vi "dfd_Calculate Size TF Polynomial.vi"(4 "alignment(left, top)":T2, 5 "format string":string="%.0f", 6 "rendering options":T1, 7 "Fonts Input":T3(array[cluster]), 8 "variable":string="s", 9 "origin":cluster{"x":i16, "y":i16}={"x"=60, "y"=30}, 10 "coefficients":dbl[](array[numeric])=[0.0, 1.0] format="%.2f") -> (2 "text rect":T4={"left"=60, "top"=30, "right"=68, "bottom"=43})   [LabVIEW 2017, in "NI_DigFilter_Process.lvlib"]
doc: "This VI allow to render Polynomials in Picture Control in ascending/descending order of coefficients, ascending/descending order of polynomial and with negative coefficients."
uses:
  <vilib>/addons/Digital Filter Design/NI_DigFilter_Process.lvlib
panel:
  in  "Fonts Defaut":T3(array[cluster])=[{"Font Name:"="Tahoma", "Size"=13, "Strikeout?"=FALSE, "Italic?"=FALSE, "Underline?"=FALSE, "Outline?"=FALSE, "Shadow?"=FALSE, "Bold?"=FALSE}, {"Font Name:"="Tahoma", "Size"=13, "Strikeout?"=FALSE, "Italic?"=FALSE, "Underline?"=FALSE, "Outline?"=FALSE, "Shadow?"=FALSE, "Bold?"=FALSE}, {"Font Name:"="Tahoma", "Size"=11, "Strikeout?"=FALSE, "Italic?"=FALSE, "Underline?"=FALSE, "Outline?"=FALSE, "Shadow?"=FALSE, "Bold?"=FALSE}]
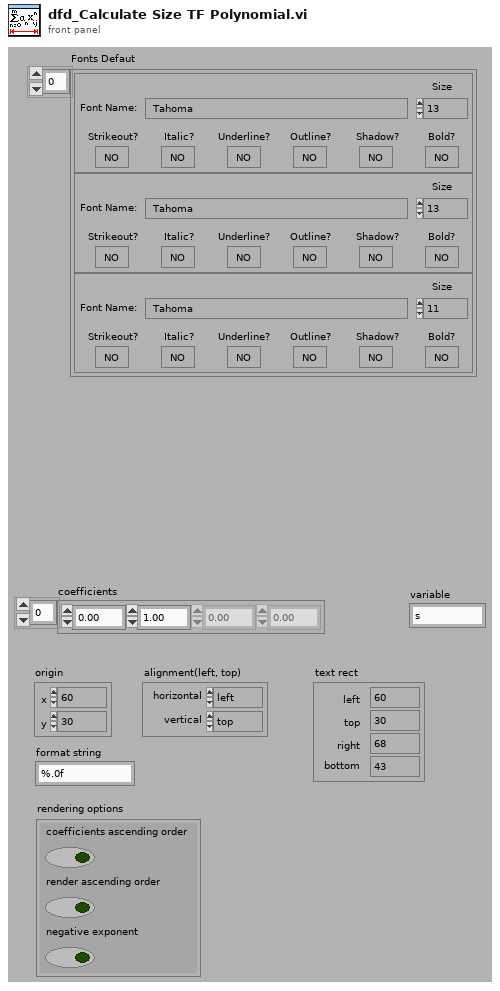
[diagram p1: front panel]
types:
  T1 = cluster{"coefficients ascending order":bool, "render ascending order":bool, "negative exponent":bool}
  T2 = cluster{"horizontal":enum16{"left", "center", "right"}, "vertical":enum16{"top", "center", "bottom"}}
  T3 = cluster{"Font Name:":string, "Size":i16, "Strikeout?":bool, "Italic?":bool, "Underline?":bool, "Outline?":bool, "Shadow?":bool, "Bold?":bool}[]
  T4 = cluster{"left":i16, "top":i16, "right":i16, "bottom":i16}
  T5 = enum16{"User-specified Font", "Application Font", "System Font", "Dialog Font"}
  T6 = cluster{"Font Name:":string, "Size":i16, "Strikeout?":bool, "Italic?":bool, "Underline?":bool, "Outline?":bool, "Shadow?":bool, "Bold?":bool}
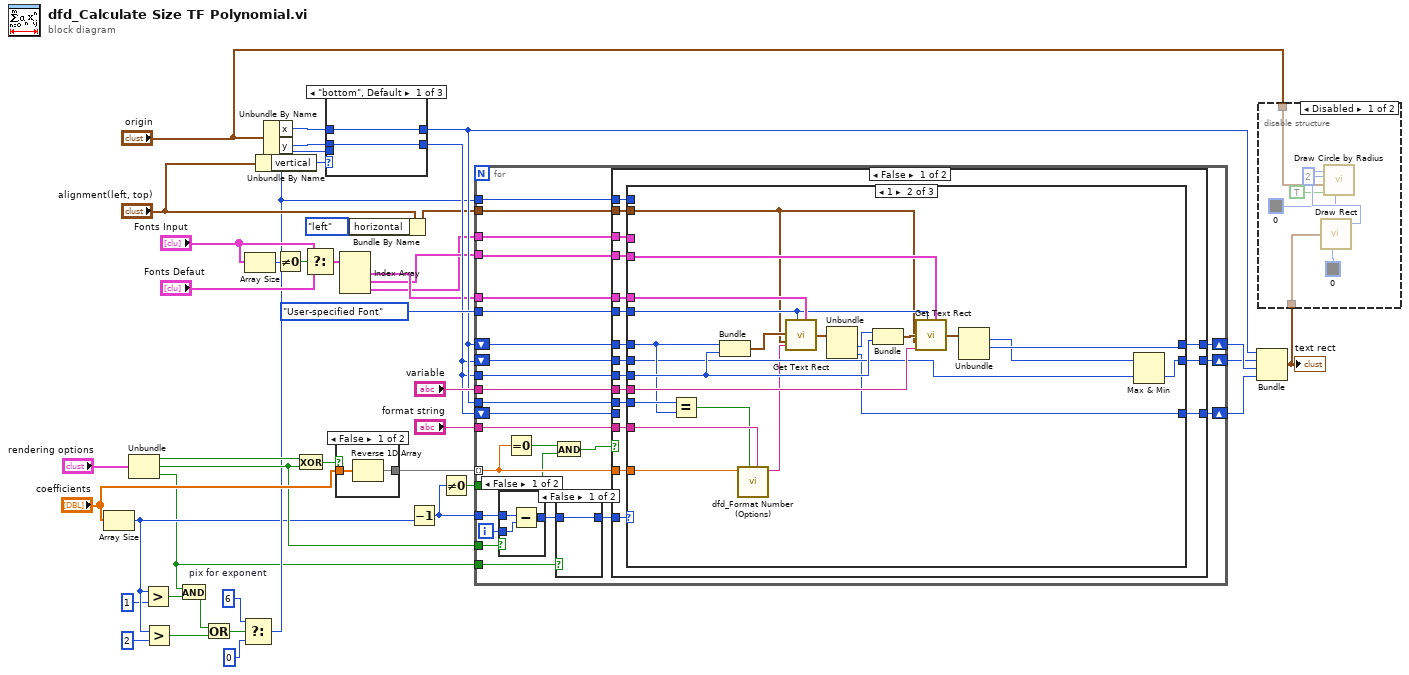
[diagram p0: block diagram]
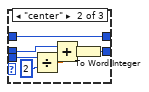
[diagram p3: hidden frame]
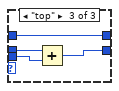
[diagram p4: hidden frame]
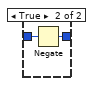
[diagram p6: hidden frame]
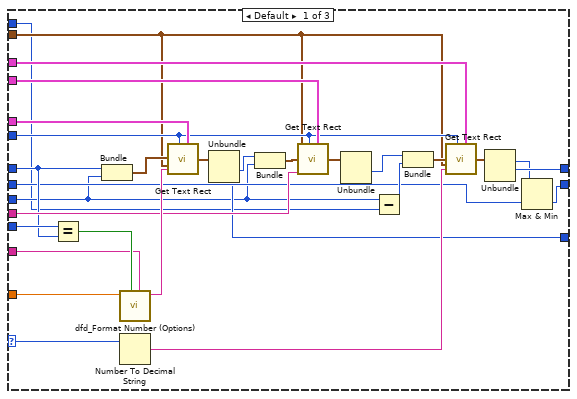
[diagram p8: hidden frame]
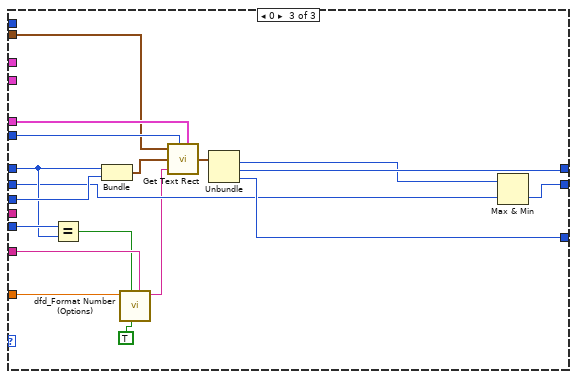
[diagram p9: hidden frame]
diagram:
  w12 = i16 6  # pix for exponent
  n1 = Array Size(array="coefficients") -> (size(s)=w5:i32)
  n2 = Unbundle("rendering options") -> ("coefficients ascending order"=w15:bool, "render ascending order"=w14:bool, "negative exponent"=w3:bool)
  n3 = Greater?(x=w5, y=1) -> (0:w2:bool)
  n4 = Greater?(x=w5, y=2) -> (0:w7:bool)
  n5 = And(x=w3, y=w2) -> (x .and. y?=w1:bool)
  n6 = Or(x=w1, y=w7) -> (x .or. y?=w6:bool)
  n7 = Select(t=w12, s=w6, f=i16 0) -> (s? t:f=w10:i16)
  n8 = Array Size(array="Fonts Input") -> (size(s)=w33:i32)
  n9 = Unbundle By Name("alignment(left, top)") -> ("vertical"=w23:enum16{"top", "center", "bottom"})
  n10 = Unbundle By Name("origin") -> ("x"=w22:i16, "y"=w21:i16)
  n11 = Not Equal To 0?(x=w33) -> (x != 0?=w34:bool)
  n12 = Exclusive Or(1:w14, 2:w15) -> (0:w25:bool)
  n13 = Select(t="Fonts Input", s=w34, f="Fonts Defaut") -> (s? t:f=w31:T3)
  n14 = case shown="\"bottom\", Default" w23 {
    tunnel: [w45 w52 w56] -> w38
    tunnel: [w44 w46 w54] -> w35
    tunnel: w22 -> [w45 w52 w56]
    tunnel: w21 -> [w44 w51 w55]
    tunnel: w10 -> [_ w49 w53]
    frame "bottom", Default {
    }
    frame "center" {
      n15 = Divide(x=w49, y=i16 2) -> (x/y=w47:dbl)
      n16 = Add(x=w51, y=w47) -> (x+y=w50:dbl)
      n17 = To Word Integer(number=w50) -> (16bit integer=w46:i16)
    }
    frame "top" {
      n18 = Add(x=w55, y=w53) -> (x+y=w54:i16)
    }
  }
  n19 = case shown="False" w25 {
    tunnel: "coefficients" -> [w58 w59]
    tunnel: [w57 w59] -> w36
    frame False {
      n20 = Reverse 1D Array(array=w58) -> (reversed array=w57:dbl[])
    }
    frame True {
    }
  }
  n21 = Index Array(array=w31) -> (element #1=w29:T6, element #2=w28:T6, element #3=w27:T6)  [unwired: 3 in]
  n22 = Bundle By Name(cluster="alignment(left, top)", "horizontal"=enum16{"left", "center", "right"}."left") -> (w19:T2)
  n23 = Decrement(x=w5) -> (x-1=w9:i32)
  n24 = Not Equal To 0?(x=w9) -> (x != 0?=w8:bool)
  n25 = for {
    tunnel: w36 -> [w68] mode=indexing
    tunnel: "variable" -> [w85]
    shift-right: [w83] -> w41
    shift-left: w38 -> [w84]
    tunnel: w35 -> [w82]
    tunnel: w29 -> [w81]
    tunnel: w27 -> [w80]
    tunnel: w28 -> [w79]
    tunnel: w38 -> [w78]
    tunnel: w9 -> [w76]
    shift-right: [w74] -> w40
    shift-left: w35 -> [w75]
    tunnel: T5."User-specified Font" ("desired font(Application)") -> [w73]
    shift-right: [w72] -> w37
    shift-left: w35 -> [w71]
    tunnel: "format string" -> [w70]
    tunnel: w19 -> [w69]
    tunnel: w14 -> [w67]
    tunnel: w3 -> [w64]
    tunnel: w10 -> [w63]
    tunnel: w8 -> [w61]
    i -> [w77]
    n26 = case shown="False" w67 {
      tunnel: w77 -> [w91 w92]
      tunnel: w76 -> [w90 _]
      tunnel: [w89 w92] -> w66
      frame False {
        n27 = Subtract(x=w90, y=w91) -> (x-y=w89:i32)
      }
      frame True {
      }
    }
    n28 = Equal To 0?(x=w68) -> (x = 0?=w60:bool)
    n29 = And(x=w60, y=w61) -> (x .and. y?=w62:bool)
    n30 = case shown="False" w64 {
      tunnel: [w86 w87] -> w65
      tunnel: w66 -> [w86 w88]
      frame False {
      }
      frame True {
        n31 = Negate(x=w88) -> (-x=w87:i32)
      }
    }
    n32 = case shown="False" w62 {
      tunnel: w85 -> [w109 _]
      tunnel: w84 -> [w108 w182]
      tunnel: [w107 w182] -> w83
      tunnel: w68 -> [w106 _]
      tunnel: w82 -> [w105 _]
      tunnel: w81 -> [w104 _]
      tunnel: w80 -> [w103 _]
      tunnel: w79 -> [w102 _]
      tunnel: w78 -> [w101 _]
      tunnel: w65 -> [w100 _]
      tunnel: w75 -> [w99 w181]
      tunnel: [w98 w181] -> w74
      tunnel: w73 -> [w97 _]
      tunnel: [w96 w180] -> w72
      tunnel: w71 -> [_ w180]
      tunnel: w70 -> [w95 _]
      tunnel: w69 -> [w94 _]
      tunnel: w63 -> [w93 _]
      frame False {
        n33 = case shown="1" w100 {
          selector: w100 -> [w111 _ _]
          tunnel: w109 -> [w125 w153 _]
          tunnel: w108 -> [w123 w151 w174]
          tunnel: [w121 w150 w173] -> w107
          tunnel: w106 -> [w113 w141 w164]
          tunnel: w105 -> [w112 w157 w176]
          tunnel: w104 -> [w132 w159 w177]
          tunnel: w103 -> [w133 _ _]
          tunnel: w102 -> [w128 w155 _]
          tunnel: w101 -> [w124 w152 w175]
          tunnel: w99 -> [w120 w149 w169]
          tunnel: [w118 w148 w167] -> w98
          tunnel: w97 -> [w117 w147 w172]
          tunnel: [w116 w146 w171] -> w96
          tunnel: w95 -> [w115 w143 w166]
          tunnel: w94 -> [w114 w145 w170]
          tunnel: w93 -> [w110 _ _]
          frame Default {
            n34 = Equal?(x=w124, y=w123) -> (x = y?=w122:bool)
            n35 = Bundle("x"=w123, "y"=w112) -> (w137:cluster{"x":i16, "y":i16})  [unwired: 1 out]
            n36 = call <vilib>:"dfd_Format Number (Options).vi"("format string"=w115, "Is Higher Coeffiecient?"=w122, "Coefficient"=w113) -> ("String Coefficient"=w139:string)  [unwired: 1 in, 7 out]
            n37 = Number To Decimal String(number=w111) -> (decimal integer string=w135:string)  [unwired: 1 out]
            n38 = call <vilib>:"Get Text Rect.vi"("alignment(left, top)"=w114, "desired font(Application)"=w117, "origin(0,0)"=w137, "text"=w139, "[user-specified font]"=w132) -> ("rect"=w138:T4)  [unwired: 1 in, 3 out]
            n39 = Unbundle(w138) -> ("right"=w127:i16, "bottom"=w116:i16)  [unwired: 2 out]
            n40 = Bundle("right"=w127, "y"=w112) -> (w131:cluster{"right":i16, "y":i16})  [unwired: 1 out]
            n41 = call <vilib>:"Get Text Rect.vi"("alignment(left, top)"=w114, "desired font(Application)"=w117, "origin(0,0)"=w131, "text"=w125, "[user-specified font]"=w128) -> ("rect"=w130:T4)  [unwired: 1 in, 3 out]
            n42 = Unbundle(w130) -> ("right"=w126:i16)  [unwired: 3 out]
            n43 = Subtract(x=w112, y=w110) -> (x-y=w134:i16)
            n44 = Bundle("right"=w126, w134) -> (w136:cluster{"right":i16, i16})  [unwired: 1 out]
            n45 = call <vilib>:"Get Text Rect.vi"("alignment(left, top)"=w114, "desired font(Application)"=w117, "origin(0,0)"=w136, "text"=w135, "[user-specified font]"=w133) -> ("rect"=w129:T4)  [unwired: 1 in, 3 out]
            n46 = Unbundle(w129) -> ("top"=w119:i16, "right"=w121:i16)  [unwired: 2 out]
            n47 = Max & Min(x=w119, y=w120) -> (min(x,y)=w118:i16)  [unwired: 1 out]
          }
          frame 1 {
            n48 = Equal?(x=w152, y=w151) -> (x = y?=w142:bool)
            n49 = Bundle("x"=w151, "y"=w157) -> (w160:cluster{"x":i16, "y":i16})  [unwired: 1 out]
            n50 = call <vilib>:"dfd_Format Number (Options).vi"("format string"=w143, "Is Higher Coeffiecient?"=w142, "Coefficient"=w141) -> ("String Coefficient"=w140:string)  [unwired: 1 in, 7 out]
            n51 = call <vilib>:"Get Text Rect.vi"("alignment(left, top)"=w145, "desired font(Application)"=w147, "origin(0,0)"=w160, "text"=w140, "[user-specified font]"=w159) -> ("rect"=w161:T4)  [unwired: 1 in, 3 out]
            n52 = Unbundle(w161) -> ("right"=w154:i16, "bottom"=w146:i16)  [unwired: 2 out]
            n53 = Bundle("right"=w154, "y"=w157) -> (w158:cluster{"right":i16, "y":i16})  [unwired: 1 out]
            n54 = call <vilib>:"Get Text Rect.vi"("alignment(left, top)"=w145, "desired font(Application)"=w147, "origin(0,0)"=w158, "text"=w153, "[user-specified font]"=w155) -> ("rect"=w156:T4)  [unwired: 1 in, 3 out]
            n55 = Unbundle(w156) -> ("top"=w144:i16, "right"=w150:i16)  [unwired: 2 out]
            n56 = Max & Min(x=w144, y=w149) -> (min(x,y)=w148:i16)  [unwired: 1 out]
          }
          frame 0 {
            n57 = Equal?(x=w175, y=w174) -> (x = y?=w165:bool)
            n58 = Bundle("x"=w174, "y"=w176) -> (w178:cluster{"x":i16, "y":i16})  [unwired: 1 out]
            n59 = call <vilib>:"dfd_Format Number (Options).vi"("format string"=w166, "Is Lower Coefficient?"=TRUE ("Is Lower Coeffiecient? 2"), "Is Higher Coeffiecient?"=w165, "Coefficient"=w164) -> ("String Coefficient"=w163:string)  [unwired: 7 out]
            n60 = call <vilib>:"Get Text Rect.vi"("alignment(left, top)"=w170, "desired font(Application)"=w172, "origin(0,0)"=w178, "text"=w163, "[user-specified font]"=w177) -> ("rect"=w179:T4)  [unwired: 1 in, 3 out]
            n61 = Unbundle(w179) -> ("top"=w168:i16, "right"=w173:i16, "bottom"=w171:i16)  [unwired: 1 out]
            n62 = Max & Min(x=w168, y=w169) -> (min(x,y)=w167:i16)  [unwired: 1 out]
          }
        }
      }
      frame True {
      }
    }
  }
  n63 = Bundle("x"=w38, "y"=w40, "x"=w41, "y"=w37) -> (w24:cluster{"x":i16, "y":i16, "x":i16, "y":i16})  [unwired: 1 out]
  "text rect" <- w24
  n64 = disable-structure shown="Disabled" {
    disable-tunnel: w24 -> [w184 _]
    disable-tunnel: "origin" -> [w183 _]
    frame Disabled {
      n65 = call <vilib>:"Draw Rect.vi"("rect"=w184, "color(black)"=u32 0) -> ("new picture"=w189:picture)  [unwired: 7 in]
      n66 = call <vilib>:"Draw Circle by Radius.vi"("color(black)"=u32 0, "fill?(F)"=TRUE, "pixel center"=w183, "radius"=i16 2, "picture"=w189) -> ()  [unwired: 6 in, 1 out]
    }
    frame Enabled {
    }
  }
